vi "Backpropagation.vi"(0 "1D ANN":i32[](array[numeric])=[4, 3, 2, 1], 1 "3D W":sgl[][][](array[numeric])=[[[1.0, 1.0, 1.0, 1.0, 1.0], [1.0, 1.0, 1.0, 1.0, 1.0], [1.0, 1.0, 1.0, 1.0, 1.0], [0.0, 0.0, 0.0, 0.0, 0.0]], [[1.0, 1.0, 1.0, 1.0, 0.0], [1.0, 1.0, 1.0, 1.0, 0.0], [0.0, 0.0, 0.0, 0.0, 0.0], [0.0, 0.0, 0.0, 0.0, 0.0]], [[1.0, 1.0, 1.0, 0.0, 0.0], [0.0, 0.0, 0.0, 0.0, 0.0], [0.0, 0.0, 0.0, 0.0, 0.0], [0.0, 0.0, 0.0, 0.0, 0.0]]] format="%.2f", 4 "Neurons outputs":sgl[][](array[numeric])=[[5.0, 5.0, 5.0, 0.0], [16.0, 16.0, 0.0, 0.0], [33.0, 0.0, 0.0, 0.0]] format="%.2f", 6 "3D W (previous)":sgl[][][](array[numeric])=[[[1.0, 1.0, 1.0, 1.0, 1.0], [1.0, 1.0, 1.0, 1.0, 1.0], [1.0, 1.0, 1.0, 1.0, 1.0], [0.0, 0.0, 0.0, 0.0, 0.0]], [[1.0, 1.0, 1.0, 1.0, 0.0], [1.0, 1.0, 1.0, 1.0, 0.0], [0.0, 0.0, 0.0, 0.0, 0.0], [0.0, 0.0, 0.0, 0.0, 0.0]], [[1.0, 1.0, 1.0, 0.0, 0.0], [0.0, 0.0, 0.0, 0.0, 0.0], [0.0, 0.0, 0.0, 0.0, 0.0], [0.0, 0.0, 0.0, 0.0, 0.0]]] format="%.2f", 8 "Function":enum16{"Linear", "Sigmoid", "Tangent hyp."}(ring), 9 "Inputs":sgl[](array[numeric])=[1.0, 1.0, 1.0, 1.0] format="%.2f", 10 "Learn rate":sgl format="%.6f", 11 "Targets":sgl[](array[numeric])=[1.0] format="%.2f", 12 "Momentum":sgl format="%.6f") -> (16 "3D updated W":sgl[][][](array[numeric]) format="%.4f")   [LabVIEW 2010]
doc: "I think I have made the backprop. working. Now the weights need to be updated and the training loop added... Good luck mate..."
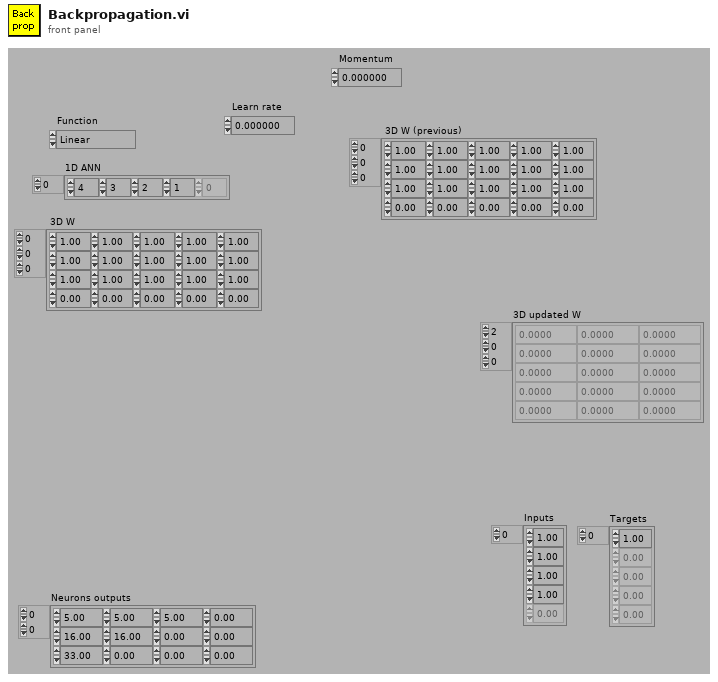
[diagram p1: front panel]
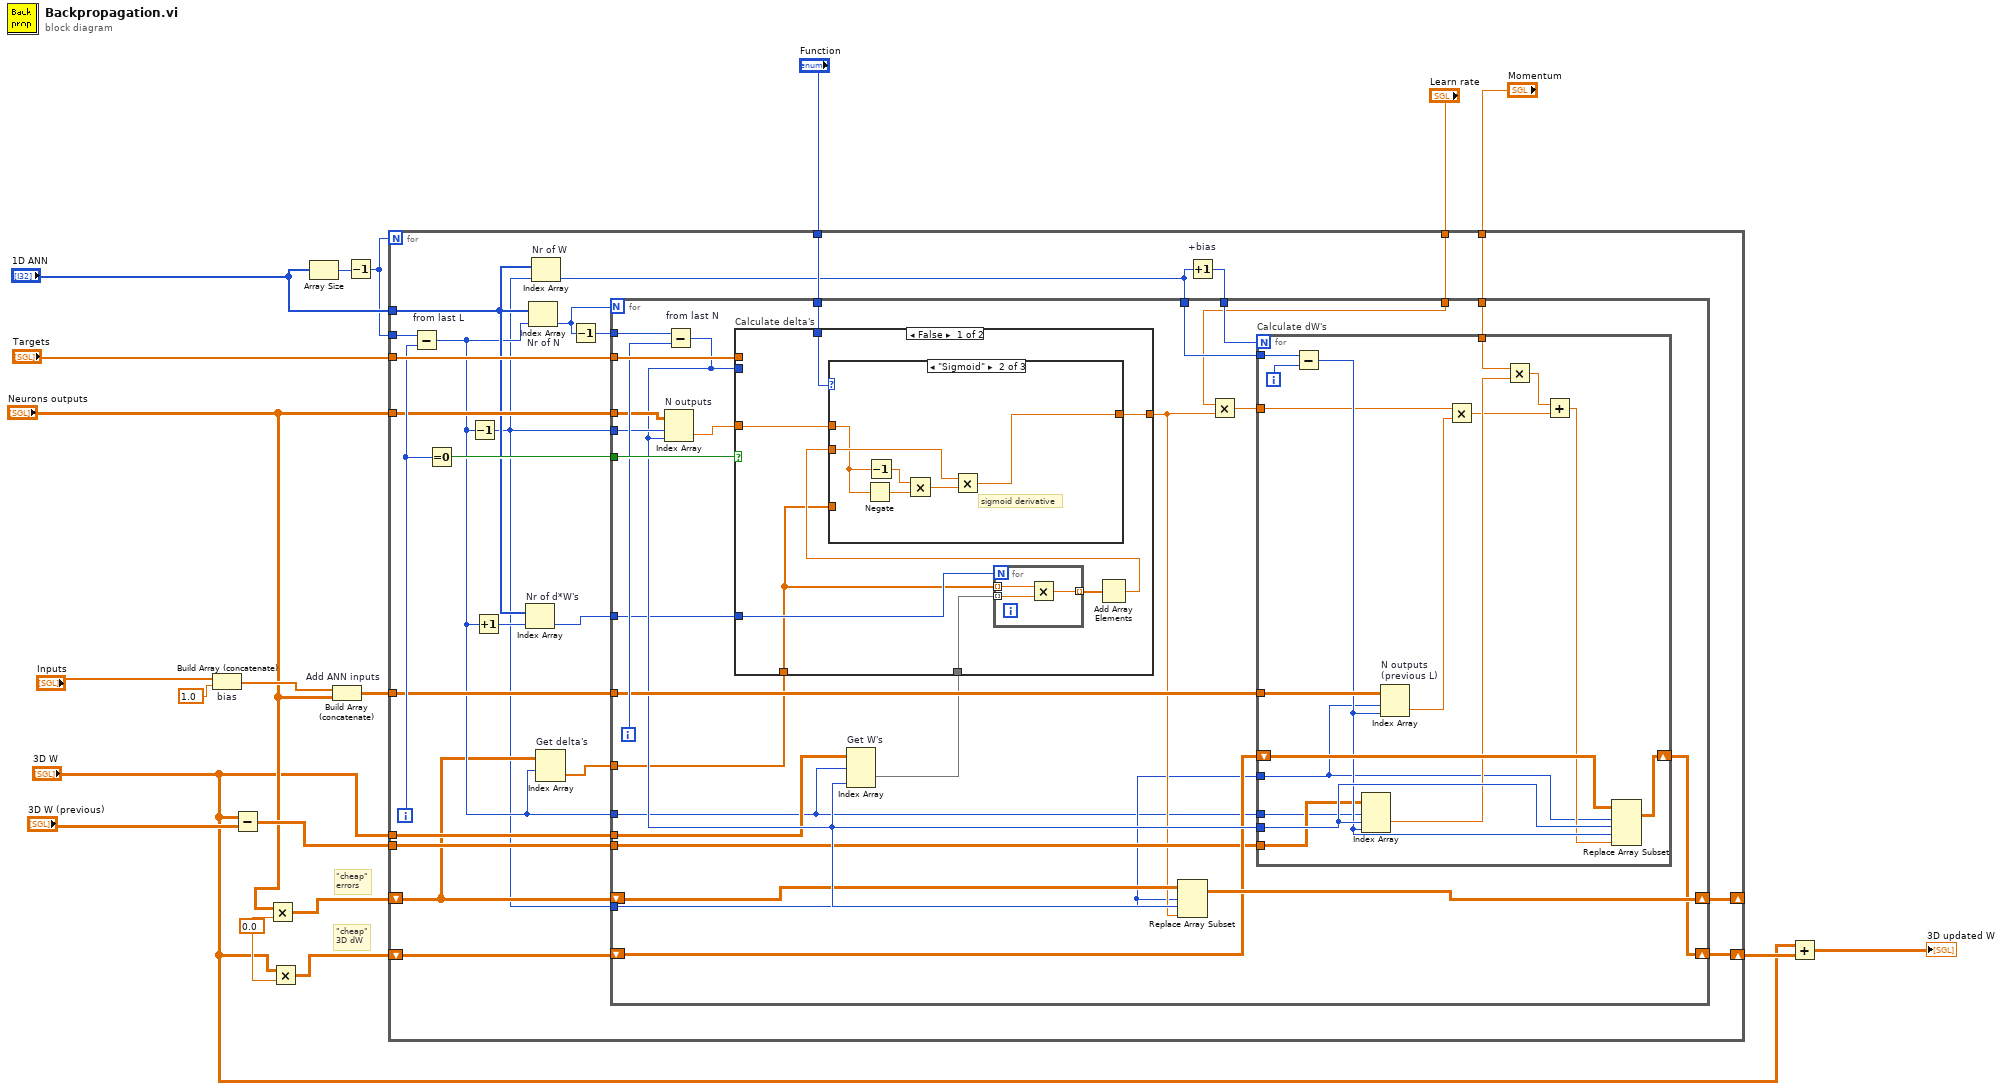
[diagram p0: block diagram]
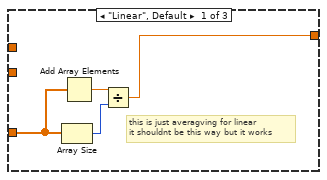
[diagram p2: hidden frame]
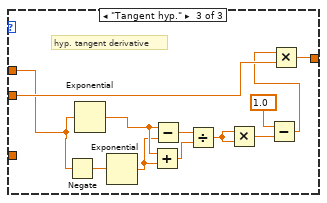
[diagram p3: hidden frame]
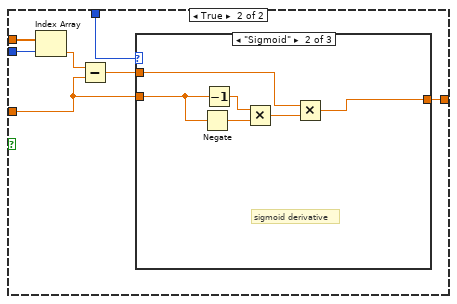
[diagram p4: hidden frame]
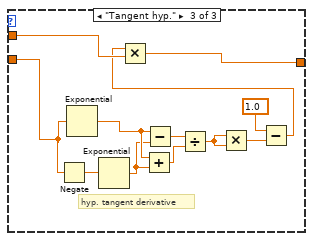
[diagram p6: hidden frame]
diagram:
  w5 = sgl 0.0
  # "\"cheap\"\nerrors"
  # "\"cheap\"\n3D dW"
  n1 = Build Array (concatenate) "bias"("Inputs", sgl 1.0 ("Input Element")) -> (w11:sgl[])
  n2 = Subtract(x="3D W", y="3D W (previous)") -> (x-y=w8:sgl[][][])
  n3 = Multiply(x="Neurons outputs", y=w5) -> (x*y=w3:sgl[][])
  n4 = Multiply(x="3D W", y=w5) -> (x*y=w1:sgl[][][])
  n5 = Array Size(array="1D ANN") -> (size(s)=w7:i32)
  n6 = Build Array (concatenate) "Add ANN inputs"(w11, "Neurons outputs") -> (w12:sgl[][])
  n7 = Decrement(x=w7) -> (x-1=w6:i32)
  n8 = for {
    N: w6 -> [_]
    tunnel: "Neurons outputs" -> [w37]
    tunnel: "1D ANN" -> [w27]
    tunnel: "Targets" -> [w45]
    tunnel: "Function" -> [w42]
    tunnel: "Learn rate" -> [w41]
    shift-right: [w40] -> _
    shift-left: w3 -> [w24]
    shift-right: [w39] -> w9
    shift-left: w1 -> [w38]
    tunnel: w12 -> [w36]
    tunnel: "Momentum" -> [w32]
    tunnel: "3D W" -> [w31]
    tunnel: w8 -> [w30]
    tunnel: w6 -> [w29]
    i -> [w44]
    n9 = Subtract "from last L"(x=w29, y=w44) -> (x-y=w26:i32)
    n10 = Equal To 0?(x=w44) -> (x = 0?=w43:bool)
    n11 = Decrement(x=w26) -> (x-1=w21:i32)
    n12 = Increment(x=w26) -> (x+1=w33:i32)
    n13 = Index Array "Nr of d*W's"(array=w27, index=w33) -> (element=w34:i32)
    n14 = Index Array "Nr of N"(array=w27, index=w26) -> (element=w35:i32)
    n15 = Index Array "Nr of W"(array=w27, index=w21) -> (element=w22:i32)
    n16 = Index Array "Get delta's"(array=w24, index (row)=w26) -> (element=w25:sgl[])  [unwired: 1 in]
    n17 = Decrement(x=w35) -> (x-1=w28:i32)
    n18 = Increment "+bias"(x=w22) -> (x+1=w23:i32)
    n19 = for {
      N: w35 -> [_]
      tunnel: w28 -> [w55]
      tunnel: w45 -> [w72]
      tunnel: w43 -> [w71]
      tunnel: w37 -> [w69]
      tunnel: w21 -> [w68]
      tunnel: w42 -> [w66]
      tunnel: w23 -> [w52]
      tunnel: w41 -> [w49]
      tunnel: w36 -> [w65]
      tunnel: w26 -> [w46]
      shift-right: [w62] -> w40
      shift-left: w24 -> [w53]
      shift-right: [w61] -> w39
      shift-left: w38 -> [w60]
      tunnel: w34 -> [w59]
      tunnel: w32 -> [w58]
      tunnel: w31 -> [w57]
      tunnel: w30 -> [w56]
      tunnel: w25 -> [w54]
      tunnel: w22 -> [w51]
      tunnel: w21 -> [w47]
      i -> [w70]
      n20 = Subtract "from last N"(x=w55, y=w70) -> (x-y=w64:i32)
      n21 = Index Array "N outputs"(array=w69, index (row)=w68, index (col)=w64) -> (element=w67:sgl)
      n22 = Index Array "Get W's"(array=w57, index (dim 0)=w46, index (dim 2)=w64) -> (element=w63:sgl[])  [unwired: 1 in]
      n23 = case "Calculate delta's" shown="False" w71 {
        tunnel: w72 -> [_ w129]
        tunnel: w64 -> [_ w128]
        tunnel: w67 -> [w96 w125]
        tunnel: w66 -> [w97 w126]
        tunnel: [w95 w123] -> w50
        tunnel: w54 -> [w91 _]
        tunnel: w63 -> [w90 _]
        tunnel: w59 -> [w92 _]
        frame False {
          n24 = for {
            N: w92 -> [_]
            tunnel: w91 -> [w100] mode=indexing
            tunnel: w90 -> [w99] mode=indexing
            tunnel: [w98] -> w94 mode=indexing
            n25 = Multiply(x=w100, y=w99) -> (x*y=w98:sgl)
          }
          n26 = Add Array Elements(numeric array=w94) -> (sum=w93:sgl)
          n27 = case shown="\"Sigmoid\"" w97 {
            tunnel: w96 -> [_ w105 w112]
            tunnel: w93 -> [_ w107 w121]
            tunnel: [w101 w106 w122] -> w95
            tunnel: w91 -> [w102 _ _]
            frame "Linear", Default {
              # "this is just averagving for linear\nit shouldnt be this way but it works"
              n28 = Array Size(array=w102) -> (size(s)=w104:i32)
              n29 = Add Array Elements(numeric array=w102) -> (sum=w103:sgl)
              n30 = Divide(x=w103, y=w104) -> (x/y=w101:sgl)
            }
            frame "Sigmoid" {
              # "sigmoid derivative"
              n31 = Negate(x=w105) -> (-x=w110:sgl)
              n32 = Decrement(x=w105) -> (x-1=w109:sgl)
              n33 = Multiply(x=w109, y=w110) -> (x*y=w108:sgl)
              n34 = Multiply(x=w107, y=w108) -> (x*y=w106:sgl)
            }
            frame "Tangent hyp." {
              # "hyp. tangent derivative"
              n35 = Negate(x=w112) -> (-x=w120:sgl)
              n36 = Exponential(1:w112) -> (0:w119:sgl)
              n37 = Exponential(1:w120) -> (0:w118:sgl)
              n38 = Add(x=w119, y=w118) -> (x+y=w116:sgl)
              n39 = Subtract(x=w119, y=w118) -> (x-y=w117:sgl)
              n40 = Divide(x=w117, y=w116) -> (x/y=w115:sgl)
              n41 = Multiply(x=w115, y=w115) -> (x*y=w114:sgl)
              n42 = Subtract(x=sgl 1.0, y=w114) -> (x-y=w111:sgl)
              n43 = Multiply(x=w111, y=w121) -> (x*y=w122:sgl)
            }
          }
        }
        frame True {
          n44 = Index Array(array=w129, index=w128) -> (element=w127:sgl)
          n45 = Subtract(x=w127, y=w125) -> (x-y=w124:sgl)
          n46 = case shown="\"Sigmoid\"" w126 {
            tunnel: w125 -> [_ w132 w138]
            tunnel: w124 -> [w130 w133 w147]
            tunnel: [w130 w131 w148] -> w123
            frame "Linear", Default {
            }
            frame "Sigmoid" {
              # "sigmoid derivative"
              n47 = Negate(x=w132) -> (-x=w136:sgl)
              n48 = Decrement(x=w132) -> (x-1=w135:sgl)
              n49 = Multiply(x=w135, y=w136) -> (x*y=w134:sgl)
              n50 = Multiply(x=w133, y=w134) -> (x*y=w131:sgl)
            }
            frame "Tangent hyp." {
              # "hyp. tangent derivative"
              n51 = Negate(x=w138) -> (-x=w146:sgl)
              n52 = Exponential(1:w138) -> (0:w145:sgl)
              n53 = Exponential(1:w146) -> (0:w144:sgl)
              n54 = Add(x=w145, y=w144) -> (x+y=w142:sgl)
              n55 = Subtract(x=w145, y=w144) -> (x-y=w143:sgl)
              n56 = Divide(x=w143, y=w142) -> (x/y=w141:sgl)
              n57 = Multiply(x=w141, y=w141) -> (x*y=w140:sgl)
              n58 = Subtract(x=sgl 1.0, y=w140) -> (x-y=w137:sgl)
              n59 = Multiply(x=w137, y=w147) -> (x*y=w148:sgl)
            }
          }
        }
      }
      n60 = Replace Array Subset(array=w53, new element=w50, index (row)=w47, index (col)=w64) -> (w62:sgl[][])
      n61 = Multiply(x=w49, y=w50) -> (x*y=w48:sgl)
      n62 = for "Calculate dW's" {
        N: w52 -> [_]
        tunnel: w46 -> [w74]
        tunnel: w64 -> [w86]
        tunnel: w51 -> [w78]
        tunnel: w65 -> [w88]
        shift-right: [w84] -> w61
        shift-left: w60 -> [w87]
        tunnel: w58 -> [w82]
        tunnel: w56 -> [w83]
        tunnel: w48 -> [w76]
        tunnel: w47 -> [w73]
        i -> [w89]
        n63 = Subtract(x=w78, y=w89) -> (x-y=w85:i32)
        n64 = Index Array(array=w83, index (dim 0)=w74, index (dim 1)=w86, index (dim 2)=w85) -> (element=w81:sgl)
        n65 = Index Array "N outputs\n(previous L)"(array=w88, index (row)=w73, index (col)=w85) -> (element=w77:sgl)
        n66 = Multiply(x=w76, y=w77) -> (x*y=w75:sgl)
        n67 = Multiply(x=w82, y=w81) -> (x*y=w80:sgl)
        n68 = Add(x=w80, y=w75) -> (x+y=w79:sgl)
        n69 = Replace Array Subset(array=w87, new element=w79, index (dim 0)=w73, index (dim 1)=w86, index (dim 2)=w85) -> (w84:sgl[][][])
      }
    }
  }
  n70 = Add(x="3D W", y=w9) -> (x+y=→"3D updated W":sgl[][][])
